vi "LCP Get Pump Handle.vi"(8 "error in (no error)":errorcluster caption="Fehler (Eingang, kein Fehler)", 11 "Pump Index":u8) -> (0 "error out":errorcluster caption="Fehler (Ausgang)", 3 "Pump Handle":i64)   [LabVIEW 2023, in "labbCAN_Pump_API.lvlib"]
doc: "LCP_Func dev_hdl LCP_CALL LCP_GetPumpHandle(unsigned char Index);"
uses:
  labbCAN_Pump_API.lvlib
  labbCAN_Pump_API.dll
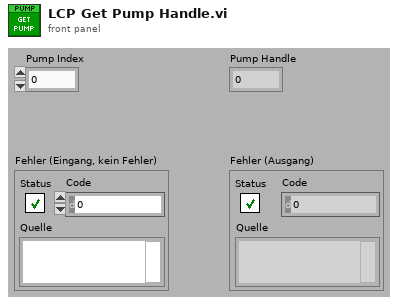
[diagram p1: front panel]
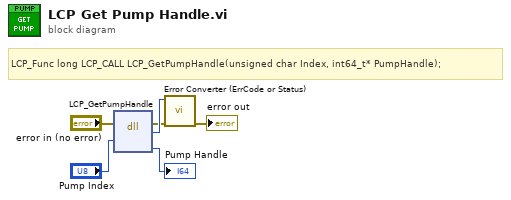
[diagram p0: block diagram]
diagram:
  # "LCP_Func long LCP_CALL LCP_GetPumpHandle(unsigned char Index, int64_t* PumpHandle);"
  n1 = dll-call lib="C:/GIT/AutomatedSetupAcousticEnergyDensity/CETONI_SDK/labbCAN_Pump_API.*" fn="LCP_GetPumpHandle"(error in="error in (no error)", "Index"="Pump Index") -> (error out=w3:errorcluster, "Rückgabetyp"=w6:i32, "PumpHandle"=→"Pump Handle":i64)  [unwired: 4 in, 1 out]
  n2 = call "Error Converter (ErrCode or Status).vi"("error in (no error)"=w3, "error code"=w6) -> ("error out"=→"error out":errorcluster)  [unwired: 9 in]
